vi "XL320_Read Motor Position.vi"(8 "error in (no error)":errorcluster, 10 "Motor ID (0)":u8, 11 "VISA resource name":refnum<visa-resource-name>) -> (0 "error out":errorcluster, 2 "Position (deg)":dbl, 3 "VISA resource name out":refnum<visa-resource-name>)   [LabVIEW 2017, in "Dynamixel XL320.lvlib"]
doc: "Reads the motor's position."
uses:
  <instrlib>/Dynamixel XL320 (Drivers instrument)/Dynamixel XL320.lvlib
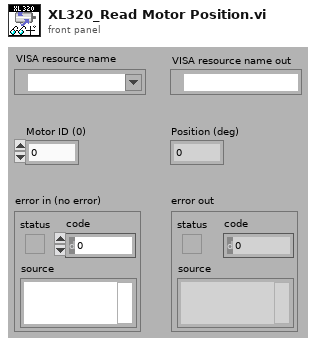
[diagram p1: front panel]
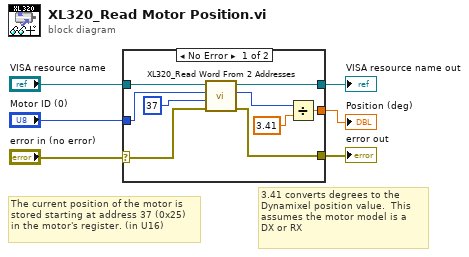
[diagram p0: block diagram]
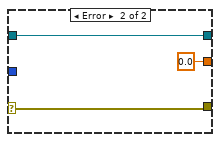
[diagram p2: hidden frame]
diagram:
  # "The current position of the motor is\nstored starting at address 37 (0x25)\nin the motor's register. (in U16)"
  # "3.41 converts degrees to the \nDynamixel position value.  This \nassumes the motor model is a \nDX or RX"
  n1 = case shown="No Error" "error in (no error)" {
    selector: "error in (no error)" -> [w10 w17]
    tunnel: "VISA resource name" -> [w13 w18]
    tunnel: [w9 w18] -> w5
    tunnel: [w7 w17] -> w4
    tunnel: [w14 0.0] -> w3
    tunnel: "Motor ID (0)" -> [w12 _]
    frame No Error {
      n2 = call <instrlib>:"XL320_Read Word From 2 Addresses.vi"("Error in (no error)"=w10, "Address number (0)"=u16 37 ("Address # DEC"), "Motor ID (0)"=w12, "VISA resource name"=w13) -> ("error out"=w7:errorcluster, "Data"=w8:u16, "VISA resource name out"=w9:refnum<visa-resource-name>)  [unwired: 5 in]
      n3 = Divide(x=w8, y=3.41) -> (x/y=w14:dbl)
    }
    frame Error {
    }
  }
  "VISA resource name out" <- w5
  "error out" <- w4
  "Position (deg)" <- w3
